vi "override.vi"(1 "Regualer":dbl, 2 "Override":bool, 3 "Invert":bool, 4 "Overriden":dbl) -> (0 "Output":dbl)   [LabVIEW 2011]
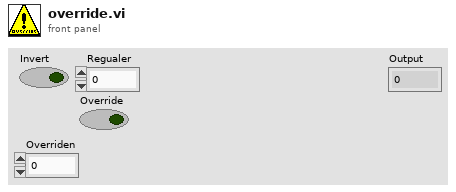
[diagram p1: front panel]
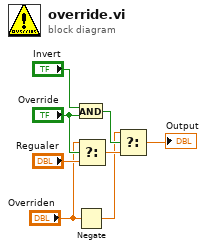
[diagram p0: block diagram]
diagram:
  n1 = And(x="Invert", y="Override") -> (x .and. y?=w4:bool)
  n2 = Negate(x="Overriden") -> (-x=w2:dbl)
  n3 = Select(t="Overriden", s="Override", f="Regualer") -> (s? t:f=w8:dbl)
  n4 = Select(t=w2, s=w4, f=w8) -> (s? t:f=→"Output":dbl)
